vi "Is not -1.vi"(4 "Number":i32) -> (1 "is not -1":bool)   [LabVIEW 2020]
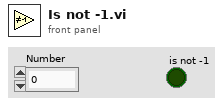
[diagram p1: front panel]
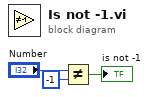
[diagram p0: block diagram]
diagram:
  n1 = Not Equal?(x="Number", y=-1) -> (x != y?=→"is not -1":bool)
